vi "GUI Show Not Available Attribute Message.vi"(5 "SGUI info control label (none)":string, 7 "SGUI control lablels to disable (empty)":string, 10 "error in":errorcluster, 11 "disabled message (empty)":string) -> (2 "error out":errorcluster)   [LabVIEW 2020]
doc: "This will check 'disabled message'. If it's not empty, it will disable SGUI lib controls to disable and enable and fill SGUI info control with 'disabled message'. It is intended to be used as explanation message when some attribute of HW is not editable."
uses:
  varilib/varilib.lvlib
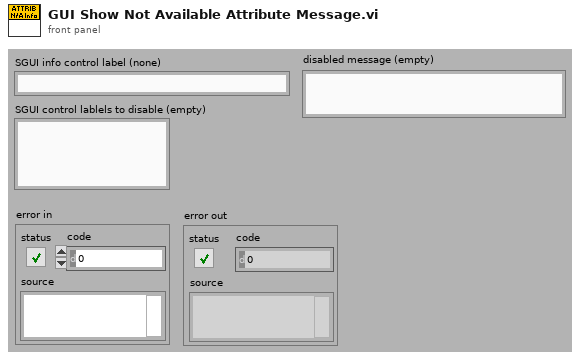
[diagram p1: front panel]
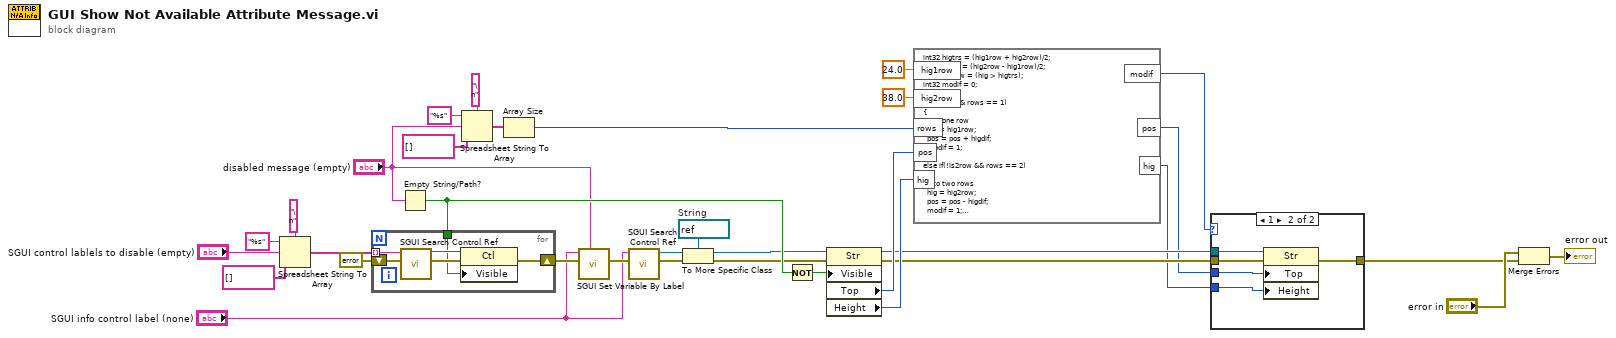
[diagram p0: block diagram]
diagram:
  w4 = refnum<vi> refnum  # String
  n1 = Spreadsheet String To Array(delimiter (Tab)="\n", format string="%s", spreadsheet string="SGUI control lablels to disable (empty)", array type (2D Dbl)=string[] []) -> (array=w31:string[])
  n2 = Empty String/Path?(string/path="disabled message (empty)") -> (empty?=w25:bool)
  n3 = for {
    tunnel: w31 -> [w40] mode=indexing
    shift-right: [w37] -> w29
    shift-left: errorcluster {"status"=FALSE, "code"=0, "source"=""} ("error out") -> [w39]
    tunnel: w25 -> [w35]
    n4 = call "SGUI Search Control Ref.vi"("error in"=w39, "control label (empty)"=w40) -> ("error out"=w38:errorcluster, "control ref out"=w36:refnum<vi>)  [unwired: 7 in, 1 out]
    n5 = property class="Ctl"(reference=w36, error in=w38, "Visible"=w35) -> (error out=w37:errorcluster)  [unwired: 1 out]
  }
  n6 = Spreadsheet String To Array(delimiter (Tab)="\n", format string="%s", spreadsheet string="disabled message (empty)", array type (2D Dbl)=string[] []) -> (array=w17:string[])
  n7 = Array Size(array=w17) -> (size(s)=w14:i32)
  n8 = call "SGUI Set Variable By Label.vi"("value (none)"="disabled message (empty)", "error in"=w29, "control label (none)"="SGUI info control label (none)") -> ("error out"=w28:errorcluster)  [unwired: 7 in, 1 out]
  n9 = call "SGUI Search Control Ref.vi"("error in"=w28, "control label (empty)"="SGUI info control label (none)") -> ("error out"=w2:errorcluster, "control ref out"=w5:refnum<vi>)  [unwired: 7 in, 1 out]
  n10 = To More Specific Class(target class=w4, reference=w5, error in=w2) -> (specific class reference=w3:refnum<vi>, error out=w1:errorcluster)
  n11 = Not(x=w25) -> (.not. x?=w26:bool)
  n12 = property class="Str"(reference=w3, error in=w1, "Visible"=w26) -> (reference out=w10:refnum<vi>, error out=w11:errorcluster, "Top"=w16:i32, "Height"=w15:u32)
  n13 = formula code="int32 higtrs = (hig1row + hig2row)/2;\nint32 higdif = (hig2row - hig1row)/2;\nint32 is2row = (hig > higtrs);\nint32 modif = 0;\n\nif(is2row && rows == 1)\n{\n  // to one row\n  hig = hig1row;\n  pos = pos + higdif;\n  modif = 1;\n}\nelse if(!is2row && rows == 2)\n{\n  // to two rows\n  hig = hig2row;\n  pos = pos - higdif;\n  modif = 1;\n}"("pos"=w16, "hig"=w15, "rows"=w14, "hig1row"=24.0 ("input variable"), "hig2row"=38.0 ("input variable")) -> ("modif"=w7:i32, "pos"=w9:i32, "hig"=w8:u32)
  n14 = case shown="1" w7 {
    tunnel: w11 -> [w41 w46]
    tunnel: w10 -> [_ w45]
    tunnel: w9 -> [_ w44]
    tunnel: w8 -> [_ w43]
    tunnel: [w41 w42] -> w6
    frame Default {
    }
    frame 1 {
      n15 = property class="Str"(reference=w45, error in=w46, "Top"=w44, "Height"=w43) -> (error out=w42:errorcluster)  [unwired: 1 out]
    }
  }
  n16 = Merge Errors("error in", w6) -> (→"error out":errorcluster)
